vi "GetType.vi"(8 "error in (no error)":errorcluster, 11 "Clear Arbitrary Sequence [SEQ] Msg":refnum<class "Clear Arbitrary Sequence [SEQ] Msg.lvclass">) -> (0 "error out":errorcluster, 2 "Data Sample":variant, 3 "Clear Arbitrary Sequence [SEQ] Msg":refnum<class "Clear Arbitrary Sequence [SEQ] Msg.lvclass">)   [LabVIEW 2015, in "CS++Fgen.lvlib" / "Clear Arbitrary Sequence [SEQ] Msg.lvclass"]
doc: "This VI delivers a sample of the data type format the message expects."
uses:
  Clear Arbitrary Sequence [SEQ] Msg.lvclass
  Clear Arbitrary Sequence [SEQ] Msg.lvclass/Clear Arbitrary Sequence [SEQ] Msg.ctl
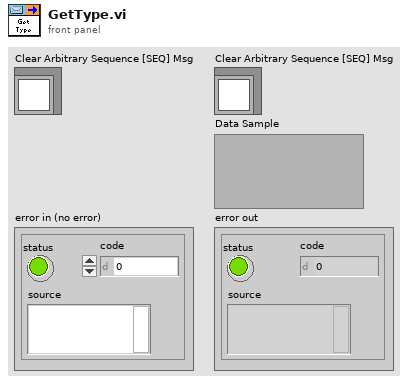
[diagram p1: front panel]
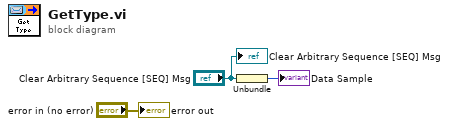
[diagram p0: block diagram]
diagram:
  n1 = Unbundle("Clear Arbitrary Sequence [SEQ] Msg") -> (→"Data Sample":i32)
  "error out" <- "error in (no error)"
  "Clear Arbitrary Sequence [SEQ] Msg" <- "Clear Arbitrary Sequence [SEQ] Msg"
